vi "acquireValue.vi"(8 "error in (no error)":errorcluster, 10 "nextSample?":bool, 11 "internalStatus in":refnum<class "internalStatus.lvclass">) -> (0 "error out":errorcluster, 1 "function return":i32, 2 "variantData":variant, 3 "internalStatus out":refnum<class "internalStatus.lvclass">)   [LabVIEW 2016, in "SALLV_AtDome_Messaging.lvlib" / "internalStatus.lvclass"]
uses:
  internalStatus.lvclass
  ts_sallv_AtDome/SALLV_AtDome.lvlib
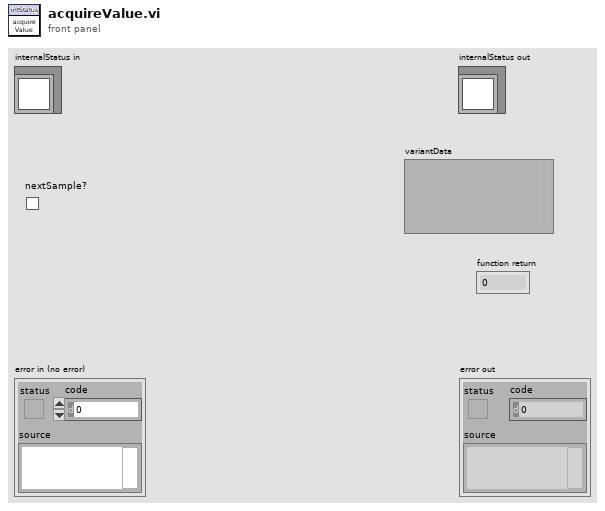
[diagram p1: front panel]
types:
  T1 = typedef "SALLV_AtDome.lvlib/logevent_internalStatus.ctl" = cluster{"code":i32, "priority":i32}
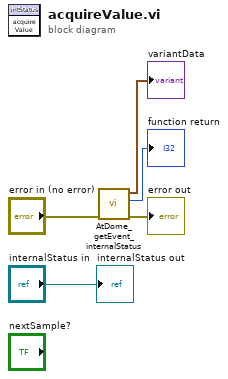
[diagram p0: block diagram]
diagram:
  n1 = call "AtDome_getEvent_internalStatus.vi"("error in (no error)"="error in (no error)") -> ("error out"=→"error out":errorcluster, "function return"=→"function return":i32, "logevent_internalStatus_Ctl out"=→"variantData":T1)  [unwired: 8 in]
  "internalStatus out" <- "internalStatus in"
